vi "Auto Measure.vi"(4 "error in":errorcluster, 7 "Data in":T1 {"LogStartTime" format="%<%x %.3X>T"}) -> (0 "error out":errorcluster, 2 "New Measure?":bool, 3 "Data Out":T1 {"LogStartTime" format="%<%x %.3X>T"})   [LabVIEW 2023]
uses:
  controls/UI Data.ctl
  <vilib>/NI/Modbus Library/API/Master/Modbus Master.lvclass
  LibreVNA/LibreVNA.lvclass
  <vilib>/Utility/error.llb/Trim Whitespace One-Sided.vi
panel:
  out "In Range?":bool
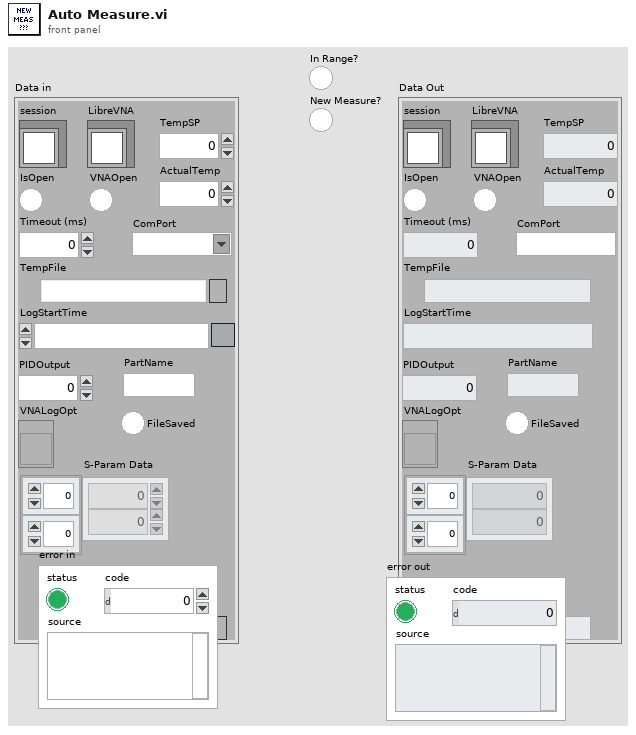
[diagram p1: front panel]
types:
  T1 = typedef "UI Data.ctl" = cluster{"session":refnum<class "Modbus Master.lvclass">, "IsOpen":bool, "Timeout (ms)":i32, "TempFile":path, "LogStartTime":timestamp, "LibreVNA":refnum<class "LibreVNA.lvclass">, "VNAOpen":bool, "TempSP":dbl, "ActualTemp":dbl, "FileSaved":bool, "PIDOutput":dbl, "VNALogOpt":refnum<vi>, "PartName":string, "ComPort":refnum<visa-resource-name>, "S-Param Data":dbl[][], "VNADataFile - TDMS":path}
  T2 = typedef "VNALogOpt.ctl" = cluster{"VNALogSelect":enum32{"No Selection", "TempIncr", "TempList"}, "VNALogTIncr":dbl, "VNALogTList":string}
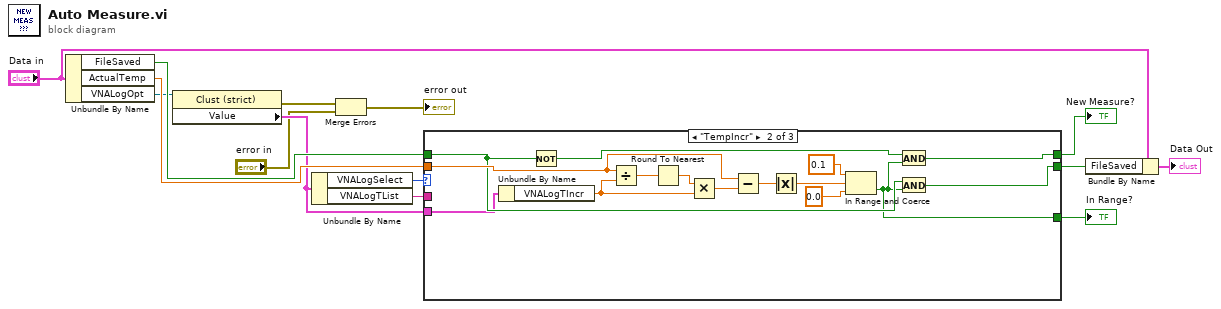
[diagram p0: block diagram]
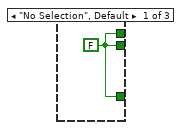
[diagram p2: hidden frame]
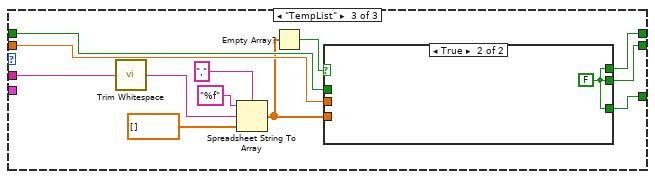
[diagram p3: hidden frame]
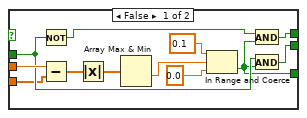
[diagram p4: hidden frame]
diagram:
  n1 = Unbundle By Name("Data in") -> ("FileSaved"=w11:bool, "ActualTemp"=w13:dbl, "VNALogOpt"=w7:refnum<vi>)
  n2 = property class="Clust (strict)"(reference=w7) -> (error out=w1:errorcluster, "Value"=w5:T2)  [unwired: 1 in, 1 out]
  n3 = Unbundle By Name(w5) -> ("VNALogSelect"=w6:enum32{"No Selection", "TempIncr", "TempList"}, "VNALogTList"=w4:string)
  n4 = Merge Errors(w1, "error in") -> (→"error out":errorcluster)
  n5 = case shown="\"TempIncr\"" w6 {
    tunnel: w13 -> [_ w28 w38]
    tunnel: [w15 w21 w37] -> w12
    tunnel: w11 -> [_ w20 w36]
    tunnel: [w15 w19 w35] -> w10
    tunnel: [w15 w18 w34] -> w8
    tunnel: w5 -> [_ w17 _]
    tunnel: w4 -> [_ _ w42]
    frame "No Selection", Default {
      w15 = FALSE
    }
    frame "TempIncr" {
      n6 = Unbundle By Name(w17) -> ("VNALogTIncr"=w16:dbl)
      n7 = Not(x=w20) -> (.not. x?=w22:bool)
      n8 = Divide(x=w28, y=w16) -> (x/y=w30:dbl)
      n9 = Round To Nearest(number=w30) -> (nearest integer value=w27:dbl)
      n10 = Multiply(x=w27, y=w16) -> (x*y=w29:dbl)
      n11 = Subtract(x=w28, y=w29) -> (x-y=w26:dbl)
      n12 = Absolute Value(x=w26) -> (abs(x)=w25:dbl)
      n13 = In Range and Coerce(upper limit=0.1, x=w25, lower limit=0.0) -> (In Range?=w19:bool)  [unwired: 1 out]
      n14 = And(x=w22, y=w19) -> (x .and. y?=w21:bool)
      n15 = And(x=w20, y=w19) -> (x .and. y?=w18:bool)
    }
    frame "TempList" {
      n16 = call <vilib>:"Trim Whitespace.vi"("string"=w42) -> ("trimmed string"=w33:string)  [unwired: 1 in]
      n17 = Spreadsheet String To Array(delimiter (Tab)=",", format string="%f", spreadsheet string=w33, array type (2D Dbl)=dbl[] []) -> (array=w32:dbl[])
      n18 = Empty Array?(array=w32) -> (empty?=w31:bool)
      n19 = case shown="True" w31 {
        tunnel: w38 -> [w54 _]
        tunnel: [w48 w55] -> w37
        tunnel: w36 -> [w46 _]
        tunnel: [w45 w55] -> w35
        tunnel: [w44 w55] -> w34
        tunnel: w32 -> [w43 _]
        frame False {
          n20 = Not(x=w46) -> (.not. x?=w47:bool)
          n21 = Subtract(x=w54, y=w43) -> (x-y=w53:dbl[])
          n22 = Absolute Value(x=w53) -> (abs(x)=w52:dbl[])
          n23 = Array Max & Min(array=w52) -> (min value=w51:dbl)  [unwired: 3 out]
          n24 = In Range and Coerce(upper limit=0.1, x=w51, lower limit=0.0) -> (In Range?=w45:bool)  [unwired: 1 out]
          n25 = And(x=w47, y=w45) -> (x .and. y?=w48:bool)
          n26 = And(x=w46, y=w45) -> (x .and. y?=w44:bool)
        }
        frame True {
          w55 = FALSE
        }
      }
    }
  }
  "In Range?" <- w10
  "New Measure?" <- w12
  n27 = Bundle By Name(cluster="Data in", "FileSaved"=w8) -> (→"Data Out":T1)
